vi "Read Processes.vi"(4 "Error In":errorcluster, 6 "Launch Condition":T1, 7 "Config Data_Text in":refnum<class "Config Data_Text.lvclass">) -> (0 "Error Out":errorcluster, 2 "Processes to Launch":T2[](array[typedef]), 3 "Config Data_Text out":refnum<class "Config Data_Text.lvclass">)   [LabVIEW 2020, in "Config Data.lvlib" / "Config Data_Text.lvclass"]
uses:
  Config Data_Text.lvclass
  typedefs/Process Launch Data.ctl
  typedefs/Process Type.ctl
  typedefs/Launch Location.ctl
  <vilib>/Utility/config.llb/Read Key (String).vi
  <vilib>/Utility/config.llb/Write Key (String).vi
  <vilib>/Utility/config.llb/NI_LVConfig.lvlib
  Config Data.lvclass
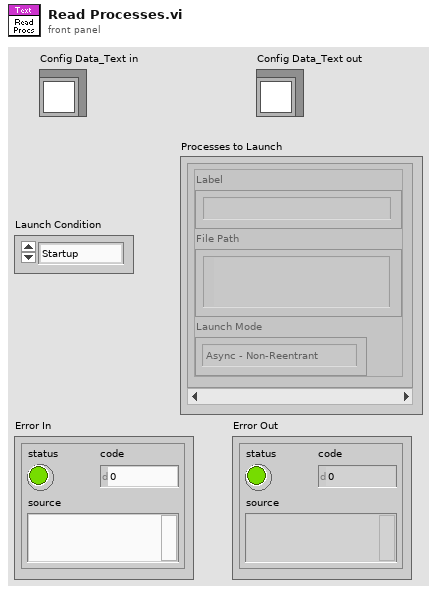
[diagram p1: front panel]
types:
  T1 = typedef "Config Data.lvlib/Config Data.lvclass/Launch Location.ctl" = enum16{"Startup", "Subpanels"}
  T2 = typedef "Config Data.lvlib/Config Data.lvclass/Process Launch Data.ctl" = cluster{"Label":string, "File Path":path, "Launch Mode":T3}
  T3 = typedef "Config Data.lvlib/Config Data.lvclass/Process Type.ctl" = enum16{"Async - Non-Reentrant", "Async - Reentrant", "Run Method - Non-Reentrant", "Run Method - Reentrant"}
  T4 = typedef "NI_LVConfig.lvlib/Config Data RefNum.ctl" = refnum<k1>
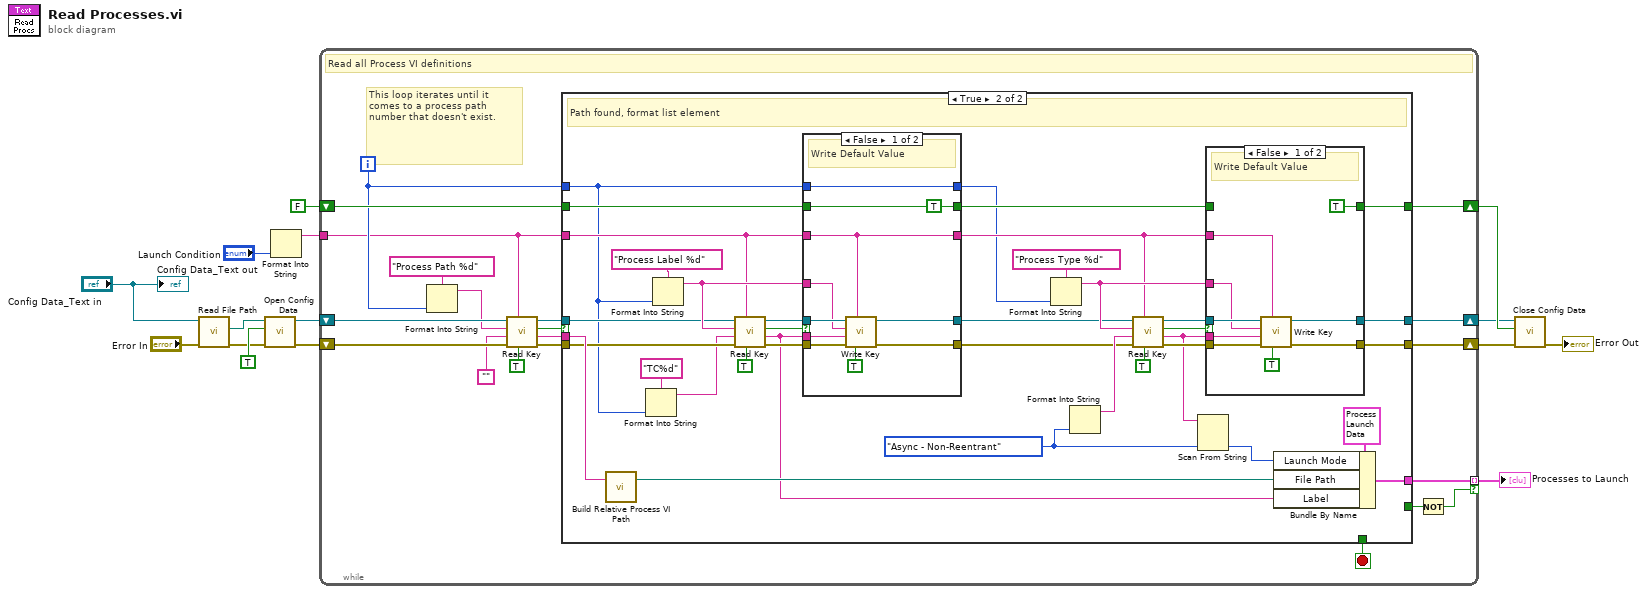
[diagram p0: block diagram]
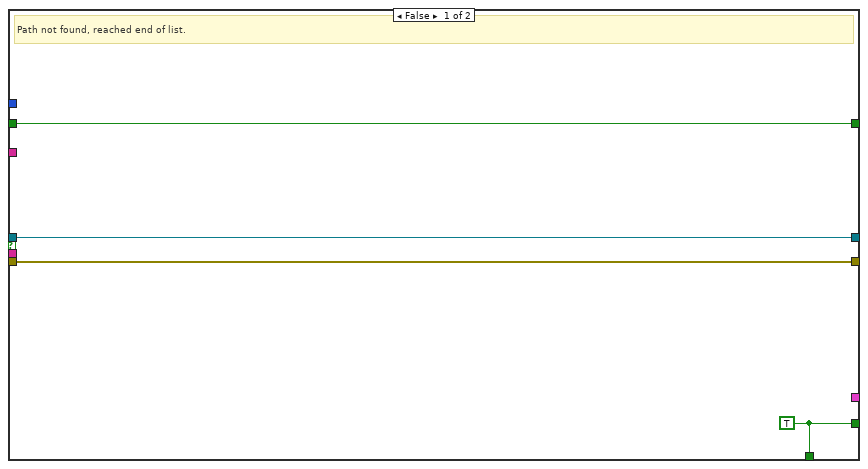
[diagram p2: hidden frame]
diagram:
  n1 = call "Read File Path.vi"("Error In"="Error In", "Text In"="Config Data_Text in") -> ("Error Out"=w3:errorcluster, "File Path"=w2:path)  [unwired: 3 in, 1 out]
  n2 = call <vilib>:"Open Config Data.vi"("error in (no error)"=w3, "create file if necessary (T)"=TRUE ("create file if necessary? (T)"), "configuration file path"=w2) -> ("error out"=w12:errorcluster, "refnum"=w11:T4)  [unwired: 6 in, 1 out]
  n3 = Format Into String("Launch Condition") -> (resulting string=w15:string)  [unwired: 3 in, 1 out]
  n4 = while {
    shift-right: [w35] -> w8
    shift-left: w11 -> [w30]
    shift-right: [w33] -> w10
    shift-left: w12 -> [w29]
    shift-right: [w34] -> w9
    shift-left: FALSE ("write configuration file? (T)") -> [w23]
    tunnel: [w19] -> w6 mode=indexing if=w18
    tunnel: w15 -> [w16]
    i -> [w20]
    stop <- w22 stop-if-true
    # "This loop iterates until it comes to a process path number that doesn't exist."
    # "Read all Process VI definitions"
    n5 = Format Into String(format string="Process Path %d" ("default value"), w20) -> (resulting string=w27:string)  [unwired: 2 in, 1 out]
    n6 = call-poly <vilib>:"Read Key.vi"("read raw string? (F)"=TRUE, "section"=w16, "error in (no error)"=w29, "default value"="", "key"=w27, "refnum"=w30) -> ("error out"=w32:errorcluster, "value"=w21:string, "found?"=w24:bool, "refnum out"=w31:T4)  [unwired: 2 out]
    n7 = case shown="True" w24 {
      tunnel: w16 -> [_ w48]
      tunnel: [w38 w74] -> w35
      tunnel: [w39 w73] -> w34
      tunnel: [w37 w72] -> w33
      tunnel: w32 -> [w37 w51]
      tunnel: w31 -> [w38 w50]
      tunnel: w23 -> [w39 w54]
      tunnel: [w36 _] -> w22
      tunnel: w21 -> [_ w70]
      tunnel: w20 -> [_ w45]
      tunnel: [_ w59] -> w19
      tunnel: [w36 _] -> w17
      frame False {
        w36 = TRUE
        # "Path not found, reached end of list."
      }
      frame True {
        w60 = Process_Type."Async - Non-Reentrant" ("Process Type")
        # "Path found, format list element"
        n8 = call "Build Relative Process VI Path.vi"("Rel Path"=w70) -> ("Full Path Out"=w58:path)  [unwired: 2 in]
        n9 = Format Into String(format string="TC%d", w45) -> (resulting string=w43:string)  [unwired: 2 in, 1 out]
        n10 = Format Into String(format string="Process Label %d" ("default value"), w45) -> (resulting string=w53:string)  [unwired: 2 in, 1 out]
        n11 = call-poly <vilib>:"Read Key.vi"("read raw string? (F)"=TRUE, "section"=w48, "error in (no error)"=w51, "default value"=w43, "key"=w53, "refnum"=w50) -> ("error out"=w52:errorcluster, "value"=w40:string, "found?"=w46:bool, "refnum out"=w55:T4)  [unwired: 2 out]
        n12 = case shown="False" w46 {
          tunnel: w55 -> [w83 w88]
          tunnel: w48 -> [w78 w86]
          tunnel: w52 -> [w84 w89]
          tunnel: [w80 w89] -> w42
          tunnel: [w81 w88] -> w41
          tunnel: w53 -> [w82 _]
          tunnel: w54 -> [_ w87]
          tunnel: [TRUE ("write configuration file? (T)") w87] -> _
          tunnel: w40 -> [w76 _]
          tunnel: [w78 w86] -> w49
          tunnel: w45 -> [w77 w85]
          tunnel: [w77 w85] -> w47
          frame False {
            # "Write Default Value"
            n13 = call-poly <vilib>:"Write Key.vi"("write raw string? (F)"=TRUE ("read raw string? (F)"), "section"=w78, "error in (no error)"=w84, "value"=w76, "key"=w82, "refnum"=w83) -> ("error out"=w80:errorcluster, "refnum out"=w81:T4)  [unwired: 4 out]
          }
          frame True {
            # "Value Found"
          }
        }
        n14 = Format Into String(format string="Process Type %d" ("default value"), w47) -> (resulting string=w64:string)  [unwired: 2 in, 1 out]
        n15 = Format Into String(w60) -> (resulting string=w61:string)  [unwired: 3 in, 1 out]
        n16 = call-poly <vilib>:"Read Key.vi"("read raw string? (F)"=TRUE, "section"=w49, "error in (no error)"=w42, "default value"=w61, "key"=w64, "refnum"=w41) -> ("error out"=w65:errorcluster, "value"=w63:string, "found?"=w68:bool, "refnum out"=w67:T4)  [unwired: 2 out]
        n17 = Scan From String(input string=w63, default 1=w60) -> (output 1=w62:T3)  [unwired: 3 in, 3 out]
        n18 = case shown="False" w68 {
          tunnel: w67 -> [w97 w100]
          tunnel: w49 -> [w96 _]
          tunnel: w65 -> [w98 w101]
          tunnel: [w93 w101] -> w72
          tunnel: [w94 w100] -> w74
          tunnel: w64 -> [w95 _]
          tunnel: w54 -> [_ w99]
          tunnel: [TRUE ("write configuration file? (T)") w99] -> w73
          tunnel: w63 -> [w91 _]
          frame False {
            # "Write Default Value"
            n19 = call-poly <vilib>:"Write Key.vi"("write raw string? (F)"=TRUE, "section"=w96, "error in (no error)"=w98, "value"=w91, "key"=w95, "refnum"=w97) -> ("error out"=w93:errorcluster, "refnum out"=w94:T4)  [unwired: 4 out]
          }
          frame True {
            # "Value Found"
          }
        }
        n20 = Bundle By Name(cluster=T2 {"Label"="", "File Path"=path "", "Launch Mode"=enum."Async - Non-Reentrant"} ("Cluster"), "Launch Mode"=w62, "File Path"=w58, "Label"=w40) -> (w59:T2)
      }
    }
    n21 = Not(x=w17) -> (.not. x?=w18:bool)
  }
  "Processes to Launch" <- w6
  n22 = call <vilib>:"Close Config Data.vi"("error in (no error)"=w10, "write file if changed (T)"=w9, "refnum"=w8) -> ("error out"=→"Error Out":errorcluster)  [unwired: 8 out]
  "Config Data_Text out" <- "Config Data_Text in"
